vi "2 Wind Records.vi"() -> ()   [LabVIEW 2011]
doc: "This VI is used by the Runprotection VI.\nSTEP 1:\nIt is evaluating the heading of the boat in comparison to the Absolute wind direction, and sets a Warning-Boolean if thos two Values get close (within a certain range).\nSTEP 2:\nIf the Warning is not active, the current wind speed and direction are logged into a global array called WindRecords. This array has a maximum size of 50. \nSTEP 2, cont'd:\nIf warning is active, the Runprotection VI is called."
uses:
  2 Typedefs/absolute wind direction.ctl
  2 Globals/2 Global.vi
panel:
  in  "Convinving Range":i32=90
  in  "Run Range":i32=15
  # "This Value is the angle in degrees from the boat to the wind,\nin which the boat counts as running."
  # "This Value sets a range, in which the VI is convinced that it is the actual wind instead of \nrandom occuring values due to running."
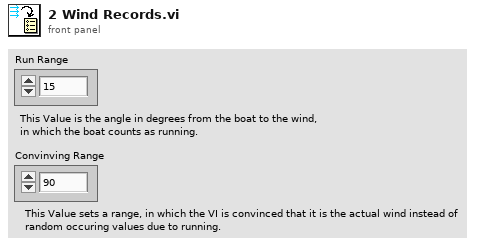
[diagram p1: front panel]
types:
  T1 = typedef "absolute wind direction.ctl" = dbl
  T2 = typedef "absolute wind speed.ctl" = dbl
  T3 = typedef "apparent wind direction.ctl" = dbl
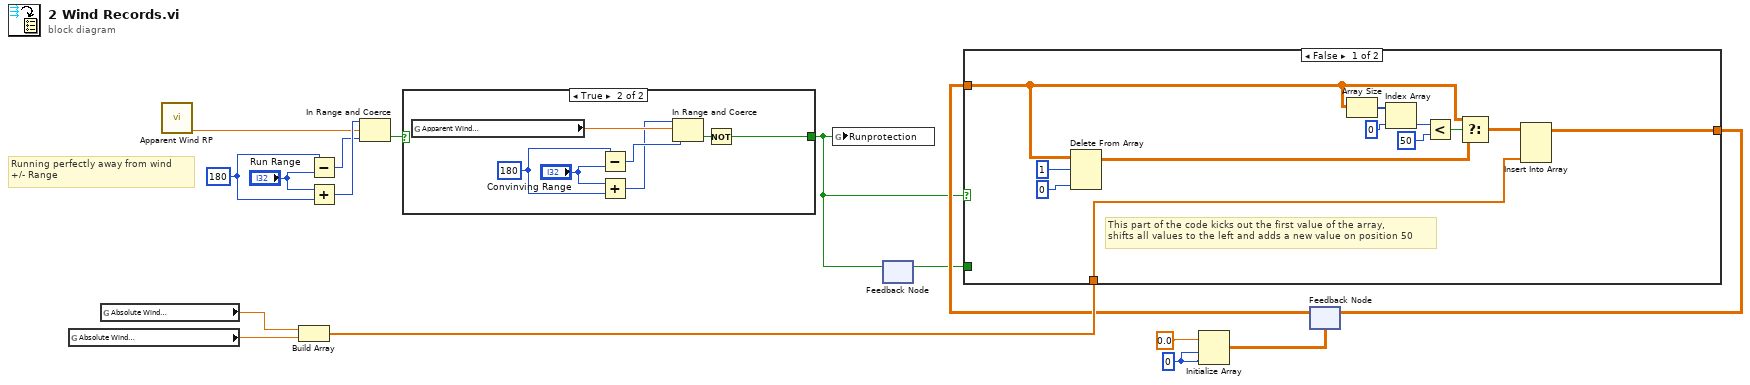
[diagram p0: block diagram]
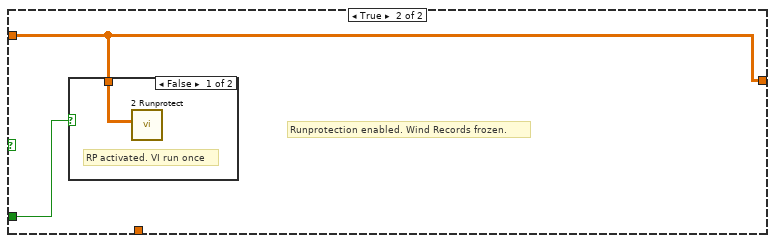
[diagram p3: hidden frame]
diagram:
  w6 = 180
  w9 = 0
  # "Running perfectly away from wind\n+/- Range"
  n1 = global read "2 Global.vi" "Absolute Wind\nDirection (º)"() -> (w15:T1)
  n2 = global read "2 Global.vi" "Absolute Wind\nSpeed"() -> (w16:T2)
  n3 = call "Apparent Wind RP.vi"() -> ("Apparent Wind Direction RP"=w3:dbl)  [unwired: 8 in, 3 out]
  n4 = Build Array(w16, w15) -> (w14:T1[])
  n5 = Subtract(x=w6, y="Run Range") -> (x-y=w4:i32)
  n6 = Add(x="Run Range", y=w6) -> (x+y=w5:i32)
  n7 = In Range and Coerce(upper limit=w5, x=w3, lower limit=w4) -> (In Range?=w2:bool)  [unwired: 1 out]
  n8 = case shown="True" w2 {
    selector: w2 -> [w17 _]
    tunnel: [w17 w23] -> w1
    frame False {
    }
    frame True {
      w21 = 180
      n9 = global read "2 Global.vi" "Apparent Wind\nDirection (º)"() -> (w22:T3)
      n10 = Subtract(x=w21, y="Convinving Range") -> (x-y=w19:i32)
      n11 = Add(x="Convinving Range", y=w21) -> (x+y=w18:i32)
      n12 = In Range and Coerce(upper limit=w18, x=w22, lower limit=w19) -> (In Range?=w24:bool)  [unwired: 1 out]
      n13 = Not(x=w24) -> (.not. x?=w23:bool)
    }
  }
  n14 = global write "2 Global.vi" "Runprotection"(w1) -> ()
  n15 = feedback #1() -> (w8:bool)  [unwired: 1 in]
  n16 = feedback-in #1(w1) -> ()
  n17 = Initialize Array(T1 0.0 ("Absolute Wind\nDirection (º)"), w9, w9) -> (w10:T1[][])
  n18 = feedback #2(w10) -> (w12:T1[][])
  n19 = case shown="False" w1 {
    tunnel: w14 -> [w36 _]
    tunnel: [w29 w38] -> w13
    tunnel: w12 -> [w28 w38]
    tunnel: w8 -> [_ w37]
    frame False {
      # "This part of the code kicks out the first value of the array, \nshifts all values to the left and adds a new value on position 50"
      n20 = Delete From Array(array=w28, length=1, index (col)=0) -> (array with subset deleted=w25:T1[][])  [unwired: 1 in, 1 out]
      n21 = Array Size(array=w28) -> (size(s)=w35:i32[])
      n22 = Index Array(array=w35, index=0) -> (element=w33:i32)
      n23 = Less?(x=w33, y=50) -> (x < y?=w31:bool)
      n24 = Select(t=w28, s=w31, f=w25) -> (s? t:f=w30:T1[][])
      n25 = Insert Into Array(array=w30, new element=w36) -> (w29:T1[][])  [unwired: 2 in]
    }
    frame True {
      # "Runprotection enabled. Wind Records frozen."
      n26 = case shown="False" w37 {
        tunnel: w38 -> [w39 _]
        frame False {
          # "RP activated. VI run once"
          n27 = call "2 Runprotect.vi"("Wind Records"=w39) -> ()  [unwired: 11 in]
        }
        frame True {
          # "Dont run it all the time"
        }
      }
    }
  }
  n28 = feedback-in #2(w13) -> ()
